vi "LabelDrag.vi"() -> ()   [LabVIEW 2012]
uses:
  <vilib>/Utility/miscctls.llb/LVPositionTypeDef.ctl
  <vilib>/Utility/miscctls.llb/LVBoundsTypeDef.ctl
  <vilib>/Utility/miscctls.llb/LVPoint32TypeDef.ctl
panel:
  out "边界 2":T1 caption="边界"
  out "时间":u32
  out "数值":i32
  out "x-y":T2
  out "位置 2":T3 caption="位置"
  out "坐标":T2 caption="鼠标按下时坐标"
  out "拖动state":bool
  in  "等待时间（毫秒）":u32=100
  in  "停止":bool
  out "二维图片":picture
  out "边界":T1
  out "位置":T3
  out "波形图":dbl[](graph)
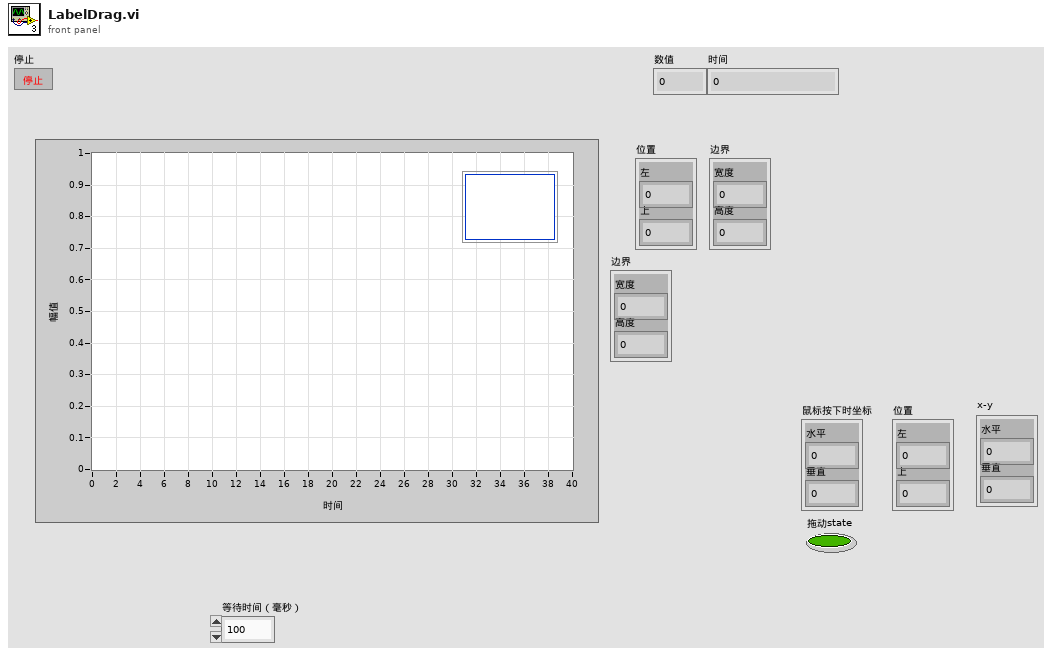
[diagram p1: front panel]
types:
  T1 = typedef "LVBoundsTypeDef.ctl" = cluster{"Width":u32, "Height":u32}
  T2 = typedef "LVPoint32TypeDef.ctl" = cluster{"Horizontal":i32, "Vertical":i32}
  T3 = typedef "LVPositionTypeDef.ctl" = cluster{"Left":i32, "Top":i32}
  T4 = cluster{"plot name":string, "plot color":u32, "fill?(F)":bool}[]
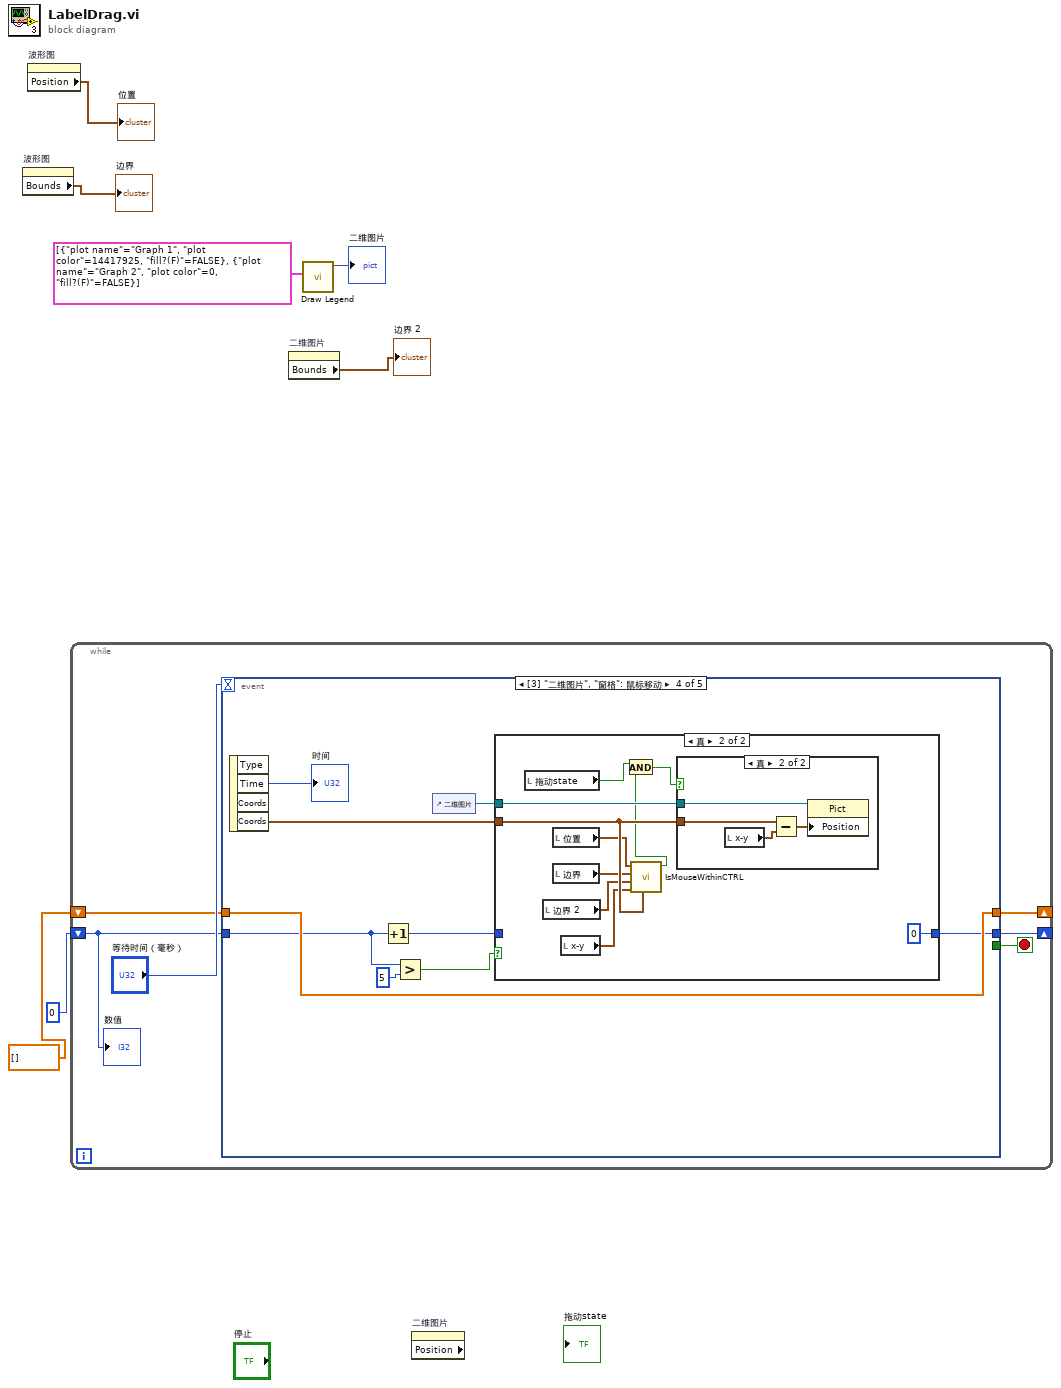
[diagram p0: block diagram]
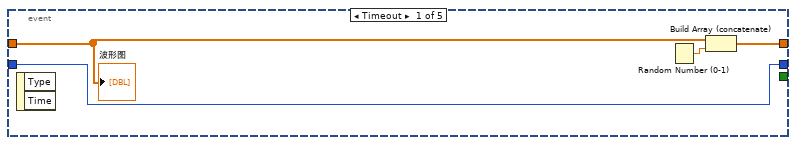
[diagram p2: hidden frame]
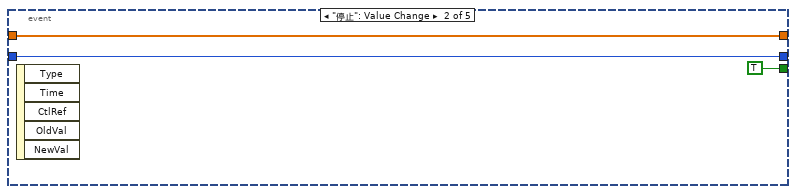
[diagram p3: hidden frame]
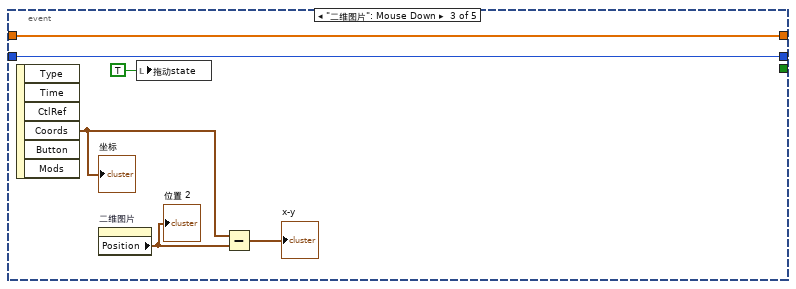
[diagram p4: hidden frame]
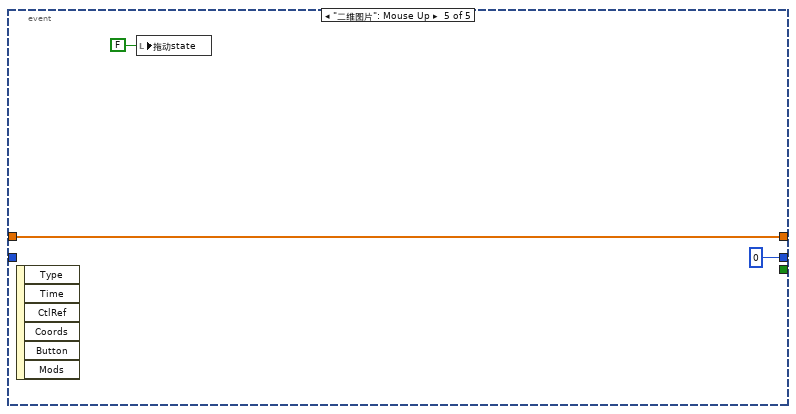
[diagram p7: hidden frame]
diagram:
  n1 = property on="波形图" class="WFGraph (严格)"() -> ("Bounds"=→"边界":T1)  [unwired: 2 in, 2 out]
  n2 = property on="波形图" class="WFGraph (严格)"() -> ("Position"=→"位置":T3)  [unwired: 2 in, 2 out]
  n3 = while {
    shift-right: [w11] -> _
    shift-left: dbl[] [] -> [w12]
    shift-right: [w8] -> _
    shift-left: 0 -> [w9]
    stop <- w10 stop-if-true
    n4 = event shown="[3] \"二维图片\", \"窗格\": 鼠标移动" {
      selector: _ -> [_ _ _ _ _]
      dyn-events: _ -> [_ _ _ _ _]
      timeout: "等待时间（毫秒）" -> [_ _ _ _ _]
      tunnel: w12 -> [w16 w19 w25 w34 w52]
      tunnel: [w15 w19 w25 w34 w52] -> w11
      tunnel: [_ TRUE _ _ _] -> w10
      tunnel: [w14 w18 w21 w32 0] -> w8
      tunnel: w9 -> [w14 w18 w21 w30 _]
      event Timeout {
        n5 = event-data() -> ()  [unwired: 1 in, 2 out]
        n6 = Random Number (0-1)() -> (number: 0 to 1=w17:dbl)
        n7 = Build Array (concatenate)(w16, w17) -> (w15:dbl[])
        "波形图" <- w16
      }
      event "停止": Value Change {
        n8 = event-data() -> ()  [unwired: 1 in, 5 out]
      }
      event "二维图片": Mouse Down {
        n9 = event-data() -> ("Coords"=w24:T2)  [unwired: 1 in, 5 out]
        "坐标" <- w24
        n10 = property on="二维图片" class="Pict"() -> ("Position"=w23:T3)  [unwired: 2 in, 2 out]
        "位置 2" <- w23
        n11 = local write "拖动state"(TRUE ("拖动state")) -> ()
        n12 = Subtract(x=w24, y=w23) -> (x-y=→"x-y":T2)
      }
      event "二维图片": Mouse Move {
        n13 = event-data() -> ("Time"=→"时间":u32, "Coords"=w35:T2)  [unwired: 1 in, 2 out]
        n14 = Increment(x=w30) -> (x+1=w29:i32)
        n15 = Greater?(x=w30, y=5) -> (0:w33:bool)
        n16 = control-ref of="二维图片"() -> (w28:refnum<vi>)
        n17 = case shown="真" w33 {
          tunnel: w28 -> [_ w46]
          tunnel: w35 -> [_ w44]
          tunnel: [w36 0 ("y")] -> w32
          tunnel: w29 -> [w36 _]
          frame False {
          }
          frame True {
            n18 = local read "拖动state"() -> (w39:bool)
            n19 = local read "边界 2"() -> (w40:T1)
            n20 = local read "位置"() -> (w42:T3)
            n21 = local read "边界"() -> (w41:T1)
            n22 = local read "x-y"() -> (w43:T2)
            n23 = call "IsMouseWithinCTRL.vi"("鼠标坐标"=w44, "x-y"=w43, "图例边界"=w40, "控件边界"=w41, "控件位置"=w42) -> ("IsMouseWithin"=w38:bool)  [unwired: 6 in]
            n24 = And(x=w39, y=w38) -> (x .and. y?=w37:bool)
            n25 = case shown="真" w37 {
              tunnel: w46 -> [_ w50]
              tunnel: w44 -> [_ w49]
              frame False {
              }
              frame True {
                n26 = local read "x-y"() -> (w48:T2)
                n27 = Subtract(x=w49, y=w48) -> (x-y=w47:T2)
                n28 = property class="Pict"(reference=w50, "Position"=w47) -> ()  [unwired: 1 in, 2 out]
              }
            }
          }
        }
      }
      event "二维图片": Mouse Up {
        n29 = event-data() -> ()  [unwired: 1 in, 6 out]
        n30 = local write "拖动state"(FALSE ("拖动state")) -> ()
      }
    }
    "数值" <- w9
  }
  n31 = property on="二维图片" class="Pict"() -> ("Bounds"=→"边界 2":T1)  [unwired: 2 in, 2 out]
  n32 = call <vilib>:"Draw Legend.vi"("plot info"=T4 [{"plot name"="Graph 1", "plot color"=14417925, "fill?(F)"=FALSE}, {"plot name"="Graph 2", "plot color"=0, "fill?(F)"=FALSE}]) -> ("new picture"=→"二维图片":picture)  [unwired: 10 in]
  n33 = property on="二维图片" class="Pict" props=["Position"]() -> ()  [unwired: 2 in, 3 out]
